vi "Create Test Configuration.vi"() -> (0 "error out":errorcluster, 1 "Names":string[](array[string]), 2 "Line Array":T1[](array[typedef]), 3 "Module Configuration":refnum<class "J1939 configuration.lvclass">, 4 "Channels":refnum<class "TBM channel.lvclass">[](array[class]), 5 "instance identifier":string, 6 "Inverted Module Config":refnum<class "J1939 configuration.lvclass">)   [LabVIEW 2015, in "J1939 tests.lvlib"]
doc: "This VI creates a standard test configuration for other unit tests. It currently creates and adds one line with every datatype to the module configuration."
uses:
  J1939 tests.lvlib
  module/configuration/J1939 configuration.lvclass
  module/configuration/Line.ctl
  <vilib>/NI/Tag Bus Module Framework/channel/TBM channel.lvclass
  <vilib>/NI/Tag Bus Module Framework/channel/channel classification.ctl
  module/configuration/XNET Settings.ctl
  <vilib>/NI/Tag Bus/tag/tag descriptor.lvclass/tag descriptor.ctl
  module/configuration/J1939 configuration.lvclass/J1939 configuration.ctl
  module/configuration/Write XNET Settings.vi
  <vilib>/NI/Configuration Framework/serializable configuration/NISE_CEF_serializable configuration.lvclass
  <vilib>/NI/Tag Bus/tag/tag descriptor.lvclass
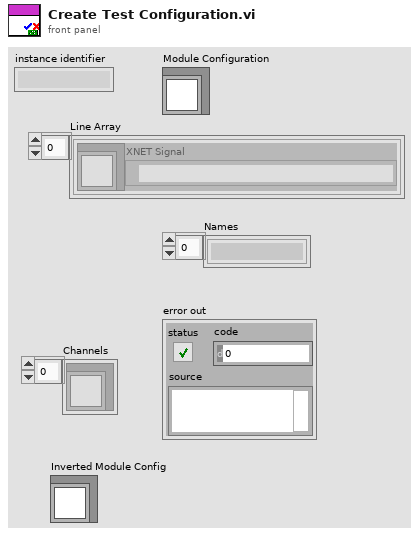
[diagram p1: front panel]
types:
  T1 = typedef "J1939 configuration.lvclass/Line.ctl" = cluster{"channel":refnum<class "TBM channel.lvclass">, "XNET Signal":refnum<k21>}
  T2 = typedef "J1939 configuration.lvclass/XNET Settings.ctl" = cluster{"Select Interface":refnum<k21>, "Claim By Adress":bool, "Node Address":u8, "Node Name":u64}
  T3 = typedef "TBM channel.lvclass/channel classification.ctl" = enum16{"input data", "output data", "processing parameter", "processing result"}
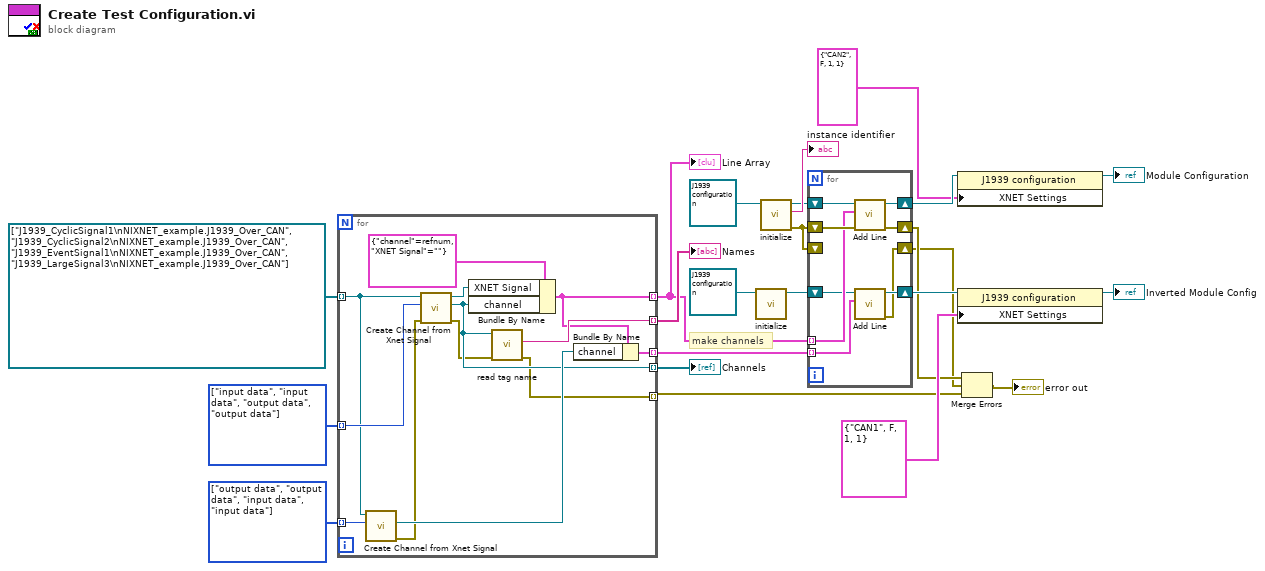
[diagram p0: block diagram]
diagram:
  w14 = T3[] [enum."output data", enum."output data", enum."input data", enum."input data"] items=["input data", "output data", "processing parameter", "processing result"]
  w15 = T3[] [enum."input data", enum."input data", enum."output data", enum."output data"] items=["input data", "output data", "processing parameter", "processing result"]
  # "make channels"
  n1 = for {
    tunnel: refnum<k21>[] ["J1939_CyclicSignal1\nNIXNET_example.J1939_Over_CAN", "J1939_CyclicSignal2\nNIXNET_example.J1939_Over_CAN", "J1939_EventSignal1\nNIXNET_example.J1939_Over_CAN", "J1939_LargeSignal3\nNIXNET_example.J1939_Over_CAN"] -> [w34] mode=indexing
    tunnel: w15 -> [w36] mode=indexing
    tunnel: w14 -> [w35] mode=indexing
    tunnel: [w30] -> w13 mode=indexing
    tunnel: [w29] -> w12 mode=indexing
    tunnel: [w28] -> w11 mode=indexing
    tunnel: [w27] -> w10 mode=indexing
    tunnel: [w24] -> w3 mode=indexing
    n2 = call "Create Channel from Xnet Signal.vi"("channel classification"=w35, "XNET Signal"=w34) -> ("error out"=w26:errorcluster, "channel"=w31:refnum<class "TBM channel.lvclass">)  [unwired: 7 in, 1 out]
    n3 = call "Create Channel from Xnet Signal.vi"("error in (no error)"=w26, "channel classification"=w36, "XNET Signal"=w34) -> ("error out"=w25:errorcluster, "channel"=w29:refnum<class "TBM channel.lvclass">, "XNET Signal 2"=w32:refnum<k21>)  [unwired: 6 in]
    n4 = Bundle By Name(cluster=T1 {"channel"=refnum, "XNET Signal"=""} ("Line"), "XNET Signal"=w32, "channel"=w29) -> (w28:T1)
    n5 = call <vilib>:"read tag name.vi"("error in"=w25, "system tag in"=w29) -> ("error out"=w24:errorcluster, "name"=w30:string)  [unwired: 7 in, 1 out]
    n6 = Bundle By Name(cluster=w28, "channel"=w31) -> (w27:T1)
  }
  "Names" <- w13
  "Line Array" <- w11
  "Channels" <- w12
  n7 = call <vilib>:"initialize.vi"("configuration in"=refnum<class "J1939 configuration.lvclass"> refnum ("tag bus configurable plugin module configuration")) -> ("configuration out"=w18:refnum<class "J1939 configuration.lvclass">)  [unwired: 8 in, 2 out]
  n8 = call <vilib>:"initialize.vi"("configuration in"=refnum<class "J1939 configuration.lvclass"> refnum ("tag bus configurable plugin module configuration")) -> ("error out"=w17:errorcluster, "identifier"=→"instance identifier":string, "configuration out"=w22:refnum<class "J1939 configuration.lvclass">)  [unwired: 8 in]
  n9 = for {
    tunnel: w11 -> [w41] mode=indexing
    shift-right: [w44] -> w21
    shift-left: w22 -> [w45]
    shift-right: [w42] -> w2
    shift-left: w17 -> [w43]
    shift-right: [w39] -> w9
    shift-left: w18 -> [w40]
    shift-right: [w38] -> w1
    shift-left: w17 -> [_]
    tunnel: w10 -> [w37] mode=indexing
    n10 = call "Add Line.vi"("error in"=w43, "Line"=w41, "J1939 configuration in"=w45) -> ("error out"=w42:errorcluster, "J1939 configuration out"=w44:refnum<class "J1939 configuration.lvclass">)  [unwired: 6 in, 1 out]
    n11 = call "Add Line.vi"("Line"=w37, "J1939 configuration in"=w40) -> ("error out"=w38:errorcluster, "J1939 configuration out"=w39:refnum<class "J1939 configuration.lvclass">)  [unwired: 7 in, 1 out]
  }
  n12 = property class="J1939 configuration"(reference=w21, "XNET Settings"=T2 {"Select Interface"="CAN2", "Claim By Adress"=FALSE, "Node Address"=1, "Node Name"=1}) -> (reference out=→"Module Configuration":refnum<class "J1939 configuration.lvclass">)  [unwired: 1 in, 1 out]
  n13 = property class="J1939 configuration"(reference=w9, "XNET Settings"=T2 {"Select Interface"="CAN1", "Claim By Adress"=FALSE, "Node Address"=1, "Node Name"=1}) -> (reference out=→"Inverted Module Config":refnum<class "J1939 configuration.lvclass">)  [unwired: 1 in, 1 out]
  n14 = Merge Errors(w2, w1, w3) -> (→"error out":errorcluster)
